vi "getDataKinect2-ElectricBoogaloo 2 - Steampunk Hullabaloo.vi"(8 "Error In":errorcluster, 10 "Image 2":T3, 11 "KinectSensor References in":T1) -> (0 "Error Out":errorcluster, 1 "Image":T3(plugin-control), 2 "Joint Position":T2, 3 "KinectSensor References":T1, 4 "Boolean":bool)   [LabVIEW 2013]
uses:
  <vilib>/MakerHub/KinectOne/KinectOne.lvlib
  <vilib>/MakerHub/KinectOne/Private/kinectRead [BodyFrame].vi
  <vilib>/MakerHub/KinectOne/Private/Type Defs/Joint Position.ctl
  <vilib>/MakerHub/KinectOne/Private/Type Defs/JointType.ctl
  <vilib>/MakerHub/KinectOne/Private/kinectRead [ColorFrame].vi
  <vilib>/MakerHub/KinectOne/Private/Type Defs/LeanTrackingState.ctl
  <vilib>/MakerHub/KinectOne/Private/Type Defs/HandRightState.ctl
  <vilib>/MakerHub/KinectOne/Private/Type Defs/HandRightConfidence.ctl
  <vilib>/MakerHub/KinectOne/Private/Type Defs/HandLeftState.ctl
  <vilib>/MakerHub/KinectOne/Private/Type Defs/HandLeftConfidence.ctl
  <vilib>/MakerHub/KinectOne/Private/Type Defs/ClippedEdges.ctl
  <vilib>/MakerHub/KinectOne/Private/Type Defs/BodyData.ctl
  Microsoft.Kinect
  C:/Program Files (x86)/National Instruments/LabVIEW 2013/vi.lib/MakerHub/KinectOne/Private/Libs/BodyFrameDataInterface.dll
  Program Files (x86)/National Instruments/LabVIEW 2013/vi.lib/MakerHub/KinectOne/Private/Libs/BodyFrameDataInterface.dll
  <vilib>/MakerHub/KinectOne/Private/Type Defs/KinectSensor References.ctl
  <vilib>/vision/Image Controls.llb/IMAQ Image.ctl
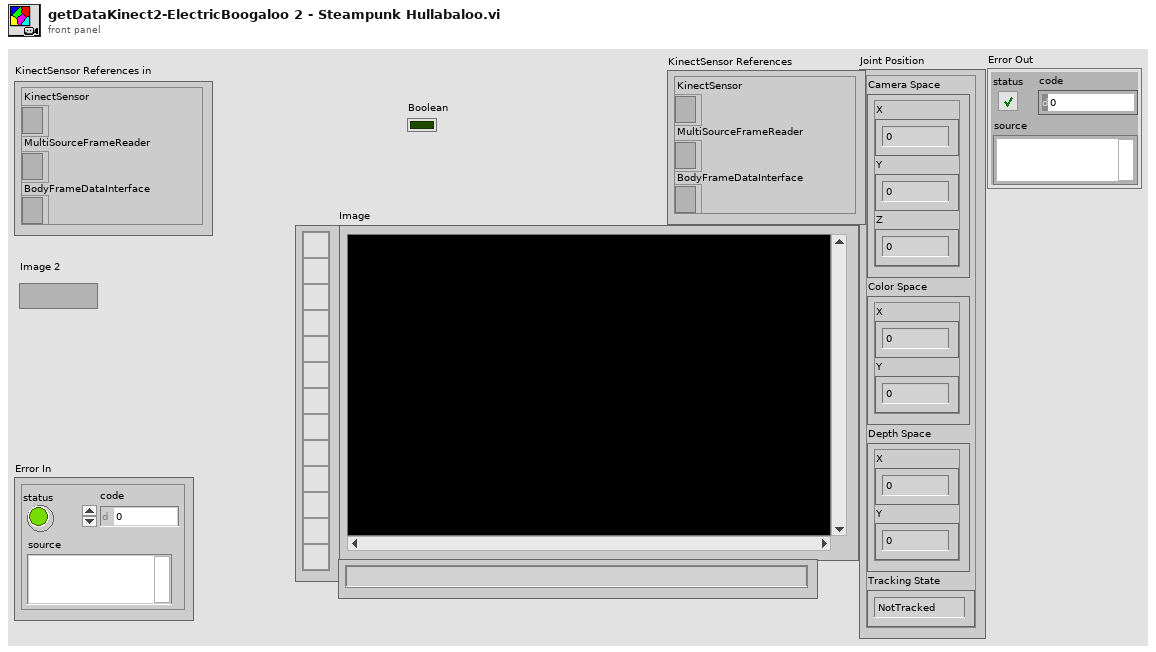
[diagram p1: front panel]
types:
  T1 = typedef "KinectOne.lvlib/KinectSensor References.ctl" = cluster{"KinectSensor":refnum<k24>, "MultiSourceFrameReader":refnum<k24>, "BodyFrameDataInterface":refnum<k24>}
  T2 = typedef "KinectOne.lvlib/Joint Position.ctl" = cluster{"Camera Space":cluster{"X":dbl, "Y":dbl, "Z":dbl}, "Color Space":cluster{"X":dbl, "Y":dbl}, "Depth Space":cluster{"X":dbl, "Y":dbl}, "Tracking State":enum16{"NotTracked", "Inferred", "Tracked"}}
  T3 = typedef "IMAQ Image.ctl" = refnum<image>
  T4 = enum16{"None Tracked", "One Tracked", "Multiple Tracked"}
  T5 = typedef "KinectOne.lvlib/BodyData.ctl" = cluster{"ClippedEdges":T6, "HandLeftConfidence":T7, "HandLeftState":T8, "HandRightConfidence":T9, "HandRightState":T10, "IsRestricted":bool, "IsTracked":bool, "JointOrientations":refnum<k24>, "Joints":refnum<k24>, "Lean":refnum<k24>, "LeanTrackingState":T11, "TrackingId":u64}
  T6 = typedef "KinectOne.lvlib/ClippedEdges.ctl" = enum16{"None", "Right", "Left", "Top", "Bottom"}
  T7 = typedef "KinectOne.lvlib/HandLeftConfidence.ctl" = enum16{"Low", "High"}
  T8 = typedef "KinectOne.lvlib/HandLeftState.ctl" = enum16{"Unknown", "NotTracked", "Open", "Closed", "Lasso"}
  T9 = typedef "KinectOne.lvlib/HandRightConfidence.ctl" = enum16{"Low", "High"}
  T10 = typedef "KinectOne.lvlib/HandRightState.ctl" = enum16{"Unknown", "NotTracked", "Open", "Closed", "Lasso"}
  T11 = typedef "KinectOne.lvlib/LeanTrackingState.ctl" = enum16{"NotTracked", "Inferred", "Tracked"}
  T12 = typedef "KinectOne.lvlib/JointType.ctl" = enum16{"SpineBase", "SpineMid", "Neck", "Head", "ShoulderLeft", "ElbowLeft", "WristLeft", "HandLeft", "ShoulderRight", "ElbowRight", "WristRight", "HandRight", "HipLeft", "KneeLeft", "AnkleLeft", "FootLeft", "HipRight", "KneeRight", "AnkleRight", "FootRight", "SpineShoulder", "HandTipLeft", "ThumbLeft", "HandTipRight", "ThumbRight"}
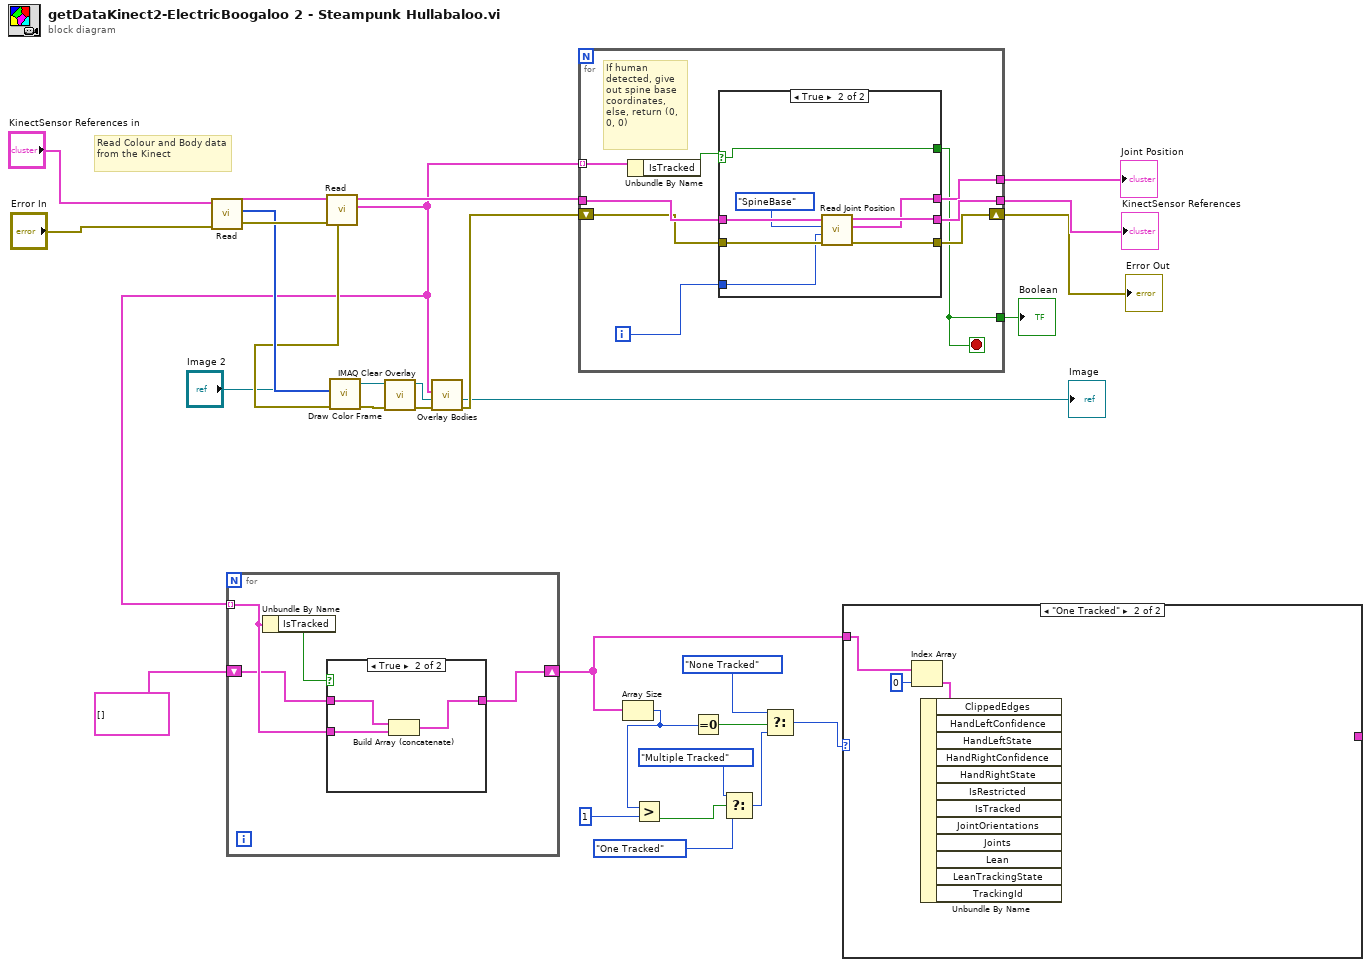
[diagram p0: block diagram]
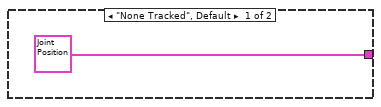
[diagram p2: hidden frame]
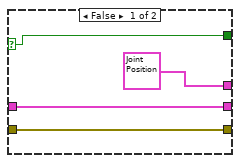
[diagram p4: hidden frame]
diagram:
  # "Read Colour and Body data from the Kinect"
  n1 = call-poly <vilib>:"Read.vi"("Error In"="Error In", "KinectSensor References in"="KinectSensor References in") -> ("Error Out"=w29:errorcluster, "frameData"=w24:u32[], "KinectSensor References out"=w28:T1)  [unwired: 7 in]
  n2 = call-poly <vilib>:"Read.vi"("error in (no error)"=w29, "KinectSensor References in"=w28) -> ("error out"=w23:errorcluster, "Body Data"=w12:T5[], "KinectSensor References out"=w30:T1)  [unwired: 7 in]
  n3 = for {
    tunnel: w12 -> [w33] mode=indexing
    shift-right: [w31] -> w1
    shift-left: T5[] [] ("Body Data") -> [w32]
    n4 = Unbundle By Name(w33) -> ("IsTracked"=w34:bool)
    n5 = case shown="True" w34 {
      tunnel: w33 -> [_ w37]
      tunnel: w32 -> [w35 w38]
      tunnel: [w35 w36] -> w31
      frame False {
      }
      frame True {
        n6 = Build Array (concatenate)(w38, w37) -> (w36:T5[])
      }
    }
  }
  n7 = call <vilib>:"Draw Color Frame.vi"("Error In"=w23, "U32 Array"=w24, "Image"="Image 2") -> ("Error Out"=w19:errorcluster, "Image Out"=w27:T3)  [unwired: 7 in]
  n8 = call "IMAQ Clear Overlay"("error in (no error)"=w19, "Image"=w27) -> ("error out"=w18:errorcluster, "Image Out"=w13:T3)  [unwired: 8 in]
  n9 = call <vilib>:"Overlay Bodies.vi"("Error In"=w18, "Image"=w13, "Body Data"=w12) -> ("Error Out"=w22:errorcluster, "Image Out"=→"Image":T3)  [unwired: 7 in]
  n10 = for {
    shift-right: [w42] -> w15
    shift-left: w22 -> [w43]
    tunnel: w12 -> [w47] mode=indexing
    tunnel: w30 -> [w46]
    tunnel: [w45] -> w16
    tunnel: [w44] -> w17
    tunnel: [w40] -> w14
    i -> [w39]
    stop <- w40 stop-if-true
    # "If human detected, give out spine base coordinates,\nelse, return (0, 0, 0)"
    n11 = Unbundle By Name(w47) -> ("IsTracked"=w41:bool)
    n12 = case shown="True" w41 {
      selector: w41 -> [w48 w55]
      tunnel: w46 -> [w51 w59]
      tunnel: [w51 w58] -> w45
      tunnel: [T2 {"Camera Space"={"X"=0.0, "Y"=0.0, "Z"=0.0}, "Color Space"={"X"=0.0, "Y"=0.0}, "Depth Space"={"X"=0.0, "Y"=0.0}, "Tracking State"=enum."NotTracked"} ("Joint Position") w56] -> w44
      tunnel: w43 -> [w49 w54]
      tunnel: [w49 w53] -> w42
      tunnel: [w48 w55] -> w40
      tunnel: w39 -> [_ w52]
      frame False {
      }
      frame True {
        n13 = call <vilib>:"Read Joint Position.vi"("Error In"=w54, "Body Index"=w52, "JointType"=JointType."SpineBase", "KinectSensor References"=w59) -> ("Error Out"=w53:errorcluster, "Joint Position"=w56:T2, "KinectSensor References"=w58:T1)  [unwired: 4 in, 1 out]
      }
    }
  }
  "Joint Position" <- w17
  "KinectSensor References" <- w16
  "Error Out" <- w15
  "Boolean" <- w14
  n14 = Array Size(array=w1) -> (size(s)=w9:i32)
  n15 = Greater?(x=w9, y=1) -> (0:w8:bool)
  n16 = Equal To 0?(x=w9) -> (x = 0?=w10:bool)
  n17 = Select(t=T4."Multiple Tracked", s=w8, f=T4."One Tracked") -> (s? t:f=w7:T4)
  n18 = Select(t=T4."None Tracked", s=w10, f=w7) -> (s? t:f=w2:T4)
  n19 = case shown="\"One Tracked\"" w2 {
    tunnel: w1 -> [_ w63]
    tunnel: [T2 {"Camera Space"={"X"=0.0, "Y"=0.0, "Z"=0.0}, "Color Space"={"X"=0.0, "Y"=0.0}, "Depth Space"={"X"=0.0, "Y"=0.0}, "Tracking State"=enum."NotTracked"} ("Joint Position") _] -> _
    frame "None Tracked", Default {
    }
    frame "One Tracked" {
      n20 = Index Array(array=w63, index=0) -> (element=w61:T5)
      n21 = Unbundle By Name(w61) -> ()  [unwired: 12 out]
    }
  }
